vi "wrtCurrent Go.vi"(6 "axis names":string[](array[string]), 8 "error in (no error)":errorcluster, 9 "Speed":dbl format="%#_13g", 10 "distances":dbl[](array[numeric]), 11 "A3200 in":refnum<class "A3200.lvclass">) -> (0 "error out":errorcluster, 3 "A3200 out":refnum<class "A3200.lvclass">)   [LabVIEW 2016, in "A3200.lvclass"]
uses:
  A3200.lvclass
  A3200.lvclass/A3200.ctl
  <userlib>/Aerotech A3200.lnk/Aerotech VIs.lvlib
panel:
  in  "taskId":i32(ring) items=["TLibrary", "T01", "T02", "T03", "T04", "T05", "T06", "T07", "T08", "T09", "T10", "T11", "T12", "T13", "T14", "T15", "T16", "T17", "T18", "T19", "T20", "T21", "T22", "T23", "T24", "T25", "T26", "T27", "T28", "T29", "T30", "T31"]
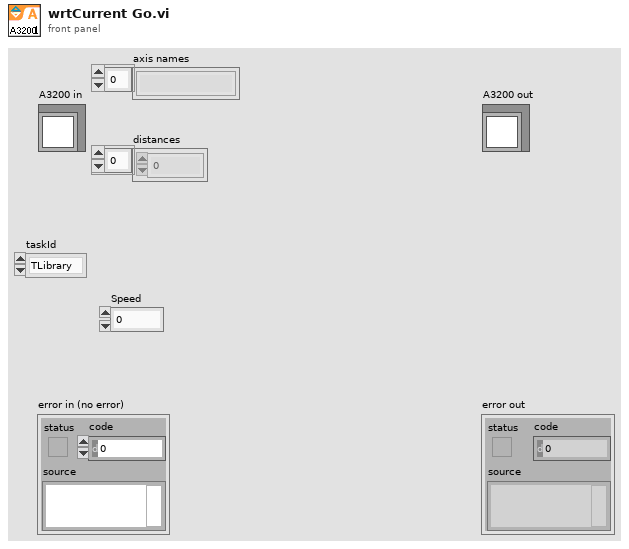
[diagram p1: front panel]
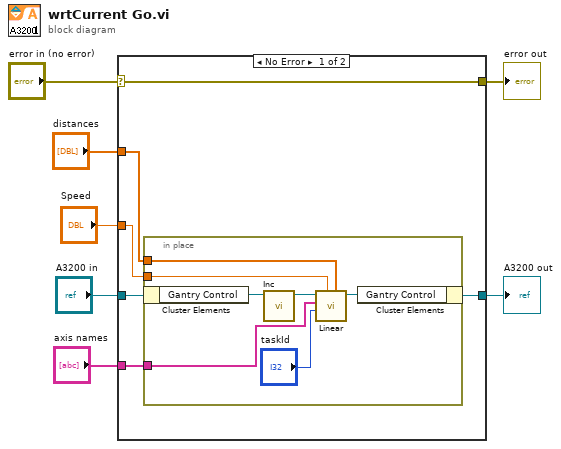
[diagram p0: block diagram]
diagram:
  n1 = case shown="No Error" "error in (no error)" {
    selector: "error in (no error)" -> [w11 w22]
    tunnel: "A3200 in" -> [w13 w21]
    tunnel: [w12 w21] -> w3
    tunnel: [w11 w22] -> w6
    tunnel: "Speed" -> [w10 _]
    tunnel: "distances" -> [w9 _]
    tunnel: "axis names" -> [w8 _]
    frame No Error {
      n2 = in-place {
        in-place-border: w10 -> [w16]
        in-place-border: w9 -> [w15]
        in-place-border: w8 -> [w14]
        n3 = in-place-cluster #1(w13) -> ("Gantry Control"=w20:refnum<k24>)
        n4 = call <userlib>:"Inc.vi"("controller in"=w20) -> ("controller out"=w19:refnum<k24>)  [unwired: 9 in, 1 out]
        n5 = call <userlib>:"Linear.vi"("distances"=w15, "speed"=w16, "taskId"="taskId", "axis names"=w14, "controller in"=w19) -> ("controller out"=w18:refnum<k24>)  [unwired: 5 in, 1 out]
        n6 = in-place-cluster #1("Gantry Control"=w18) -> (w12:refnum<class "A3200.lvclass">)
      }
    }
    frame Error {
    }
  }
  "error out" <- w6
  "A3200 out" <- w3
